vi "publishSlitWidth.vi"(8 "error in (no error)":errorcluster, 10 "position":T1, 11 "MonoCommunicator in":refnum<class "MonoCommunicator.lvclass">) -> (0 "error out":errorcluster, 3 "MonoCommunicator out":refnum<class "MonoCommunicator.lvclass">)   [LabVIEW 2016, in "MonoCommunicator.lvclass"]
uses:
  MonoCommunicator.lvclass
  Typedefs/slit.ctl
  Typedefs/SlitType.ctl
  Typedefs/slitWidth.ctl
  Typedefs/publishers.ctl
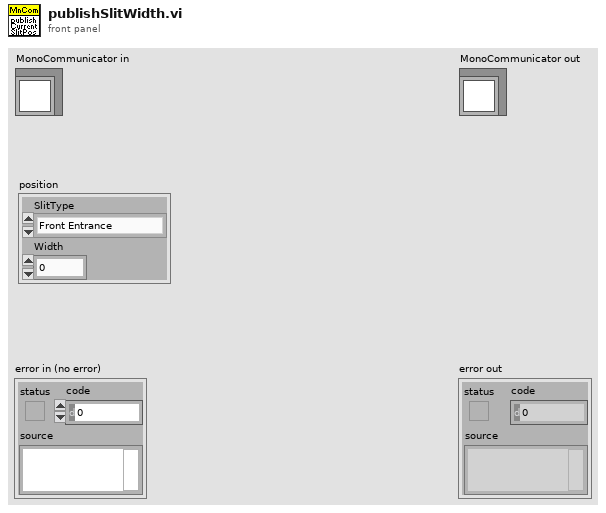
[diagram p1: front panel]
types:
  T1 = typedef "slit.ctl" = cluster{"SlitType":T2, "Width":T3}
  T2 = typedef "SlitType.ctl" = enum16{"Front Entrance", "Side Entrance", "Front Exit", "Side Exit", "First Intermediate", "Second Intermediate"}
  T3 = typedef "slitWidth.ctl" = dbl
  T4 = typedef "publishers.ctl" = enum16{"Wavelength", "Grating", "FrontEntranceSlitPosition", "FrontExitSlitPosition", "SoftwareStatus", "MonochromatorId", "Ack"}
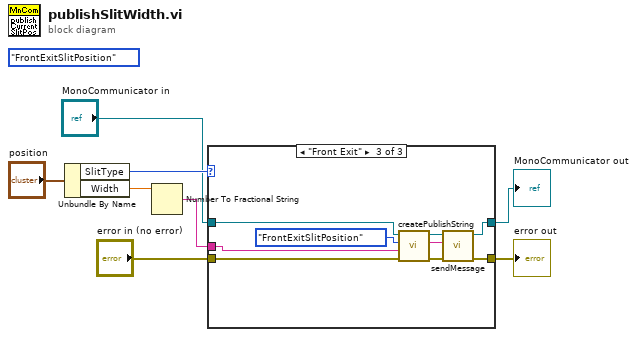
[diagram p0: block diagram]
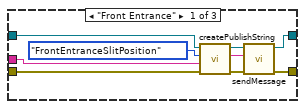
[diagram p2: hidden frame]
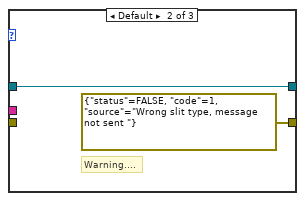
[diagram p3: hidden frame]
diagram:
  (unwired) publishers."FrontExitSlitPosition" ("publishers")
  n1 = Unbundle By Name("position") -> ("SlitType"=w7:T2, "Width"=w3:T3)
  n2 = Number To Fractional String(number=w3) -> (F-format string=w2:string)  [unwired: 3 in]
  n3 = case shown="\"Front Exit\"" w7 {
    tunnel: "error in (no error)" -> [w13 _ w27]
    tunnel: [w12 errorcluster {"status"=FALSE, "code"=1, "source"="Wrong slit type, message not sent "} ("error out") w22] -> w6
    tunnel: "MonoCommunicator in" -> [w10 w18 w28]
    tunnel: [w11 w18 w24] -> w4
    tunnel: w2 -> [w9 _ w26]
    frame "Front Entrance" {
      n4 = call "createPublishString.vi"("error in (no error)"=w13, "parameter"=w9, "publishers"=publishers."FrontEntranceSlitPosition", "MonoCommunicator in"=w10) -> ("error out"=w15:errorcluster, "string"=w16:string, "MonoCommunicator out"=w14:refnum<class "MonoCommunicator.lvclass">)  [unwired: 5 in]
      n5 = call-dynamic "sendMessage.vi"("error in (no error)"=w15, "message"=w16, "MonoCommunicator in"=w14) -> ("error out"=w12:errorcluster, "MonoCommunicator out"=w11:refnum<class "MonoCommunicator.lvclass">)  [unwired: 7 in]
    }
    frame Default {
      # "Warning...."
    }
    frame "Front Exit" {
      n6 = call "createPublishString.vi"("error in (no error)"=w27, "parameter"=w26, "publishers"=publishers."FrontExitSlitPosition", "MonoCommunicator in"=w28) -> ("error out"=w23:errorcluster, "string"=w21:string, "MonoCommunicator out"=w25:refnum<class "MonoCommunicator.lvclass">)  [unwired: 5 in]
      n7 = call-dynamic "sendMessage.vi"("error in (no error)"=w23, "message"=w21, "MonoCommunicator in"=w25) -> ("error out"=w22:errorcluster, "MonoCommunicator out"=w24:refnum<class "MonoCommunicator.lvclass">)  [unwired: 7 in]
    }
  }
  "error out" <- w6
  "MonoCommunicator out" <- w4
